vi "Contains.vi"(8 "error in (no error)":errorcluster, 9 "Item":refnum<class "ILabVIEWItem.lvclass">, 11 "CLabVIEWItem in":refnum<class "CLabVIEWItem.lvclass">) -> (0 "error out":errorcluster, 2 "Contains?":bool, 3 "CLabVIEWItem out":refnum<class "CLabVIEWItem.lvclass">)   [LabVIEW 2020, in "LabVIEWItem.lvlib" / "CLabVIEWItem.lvclass"]
uses:
  CLabVIEWItem.lvclass
  obj/Addons/LabVIEWObjectInterfaces.lvlibp/LabVIEWObjectInterfaces/ILabVIEWItem/ILabVIEWItem.lvclass
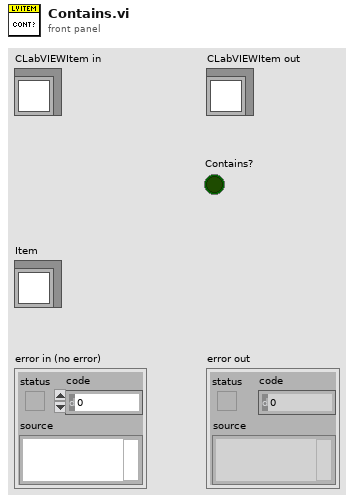
[diagram p1: front panel]
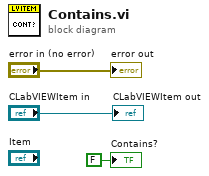
[diagram p0: block diagram]
diagram:
  "error out" <- "error in (no error)"
  "CLabVIEWItem out" <- "CLabVIEWItem in"
  "Contains?" <- FALSE ("Contains?")
